vi "Copy Definition.vi"(6 "Source Linked List ID":string, 7 "Sink Linked List ID":string, 8 "error in (no error)":errorcluster, 10 "Sink Parent Linked List ID":string, 11 "Linked List in":refnum<class "Linked List.lvclass">) -> (0 "error out":errorcluster, 3 "Linked List out":refnum<class "Linked List.lvclass">)   [LabVIEW 2017, in "Linked Lists.lvlib" / "Linked List.lvclass"]
uses:
  <vilib>/gpm_packages/@cs/linked-list/Source/Linked List/Linked List/Linked List.lvclass
  <vilib>/gpm_packages/@cs/linked-list/Source/Linked List/Linked List Definition/Linked List Definition.lvclass
  <vilib>/gpm_packages/@cs/linked-list/Source/Linked List/Linked List/Linked List.lvclass/Linked List.ctl
  <vilib>/gpm_packages/@cs/lookup-table/Source/LookupTable/LookupTable.lvclass/LookupTable.ctl
  fc44c7f0-5a9e-40d2-b54b-4ea944ea955e.vi
  566d1f49-e8c0-4e88-a1ce-2ed4a1a2aa01.vi
  d013bb3b-877c-4562-b0e2-39ea021f3923.vi
  <vilib>/gpm_packages/@cs/lookup-table/Source/LookupTable/Read Table Reference.vi
  fc44c7f0-5a9e-40d2-b54b-4ea944ea955e.vi/5b75dade-0515-45f6-8903-5eeabbbc6241.vi
  566d1f49-e8c0-4e88-a1ce-2ed4a1a2aa01.vi/ac60371e-ed5d-4c42-9a6c-bb762d6fad24.vi
  d013bb3b-877c-4562-b0e2-39ea021f3923.vi/90c978a3-e6f6-4f1a-b781-e83e293bed5b.vi
  <vilib>/gpm_packages/@cs/lookup-table/Source/LookupTable/LookupTable.lvclass
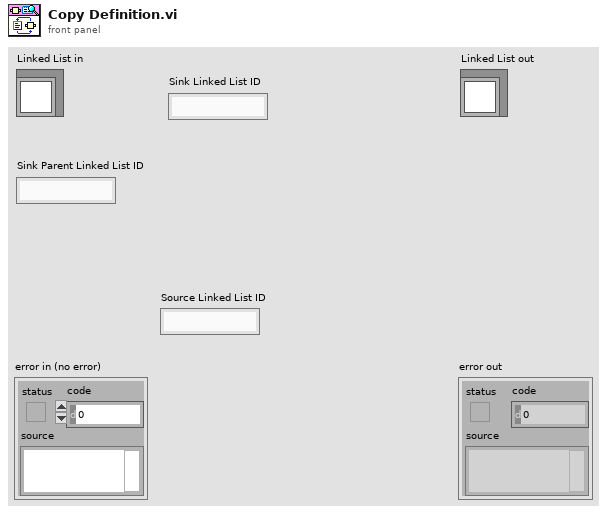
[diagram p1: front panel]
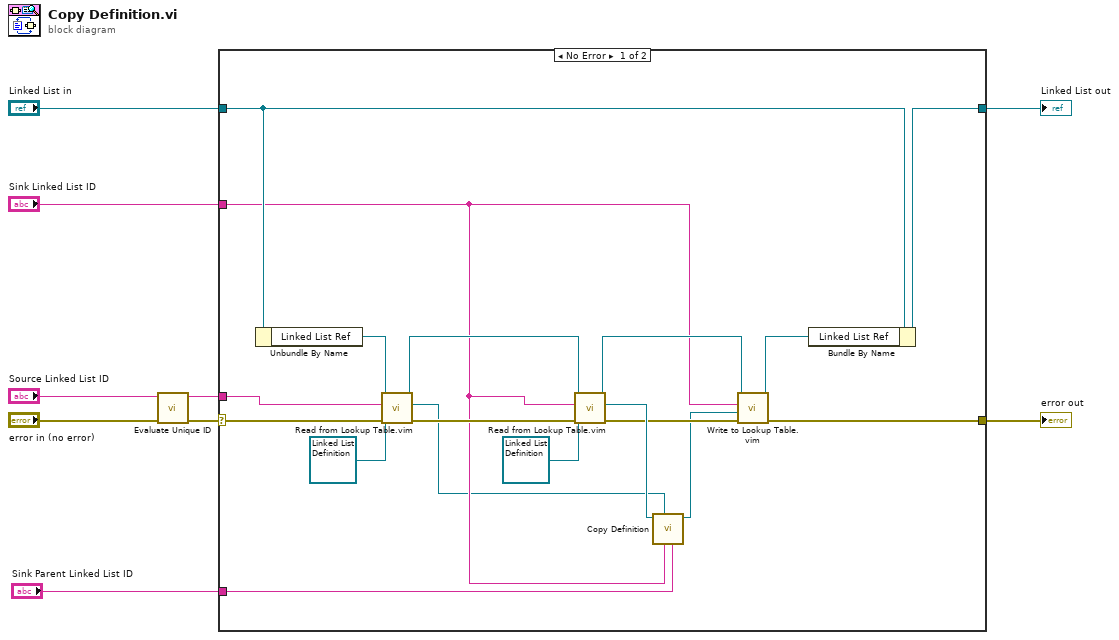
[diagram p0: block diagram]
diagram:
  n1 = call <vilib>:"Evaluate Unique ID.vi"("error in (no error)"="error in (no error)", "Unique ID"="Source Linked List ID") -> ("error out"=w5:errorcluster, "Unique ID Out"=w3:string)  [unwired: 8 in]
  n2 = case shown="No Error" w5 {
    selector: w5 -> [w25 w29]
    tunnel: [w13 w29] -> w9
    tunnel: [w22 w28] -> w7
    tunnel: "Linked List in" -> [w20 w28]
    tunnel: w3 -> [w24 _]
    tunnel: "Sink Linked List ID" -> [w12 _]
    tunnel: "Sink Parent Linked List ID" -> [w17 _]
    frame No Error {
      n3 = Unbundle By Name(w20) -> ("Linked List Ref"=w27:refnum<data-value>)
      n4 = call "Read from Lookup Table.vim"("error in (no error)"=w25, "Type"=refnum<class "Linked List Definition.lvclass"> refnum ("Linked List.lvlib:Linked List Definition.lvclass"), "Item Name"=w24, "LookupTable Reference"=w27) -> ("error out"=w21:errorcluster, "Value"=w10:refnum<class "Linked List Definition.lvclass">, "LookupTable Reference Out"=w19:refnum<data-value>)  [unwired: 4 in, 1 out]
      n5 = call "Read from Lookup Table.vim"("error in (no error)"=w21, "Type"=refnum<class "Linked List Definition.lvclass"> refnum ("Linked List.lvlib:Linked List Definition.lvclass"), "Item Name"=w12, "LookupTable Reference"=w19) -> ("error out"=w14:errorcluster, "Value"=w18:refnum<class "Linked List Definition.lvclass">, "LookupTable Reference Out"=w16:refnum<data-value>)  [unwired: 4 in, 1 out]
      n6 = call <vilib>:"Copy Definition.vi"("Parent Linked List ID"=w17, "Linked List ID"=w12, "Linked List Definition Source"=w10, "Linked List Definition in"=w18) -> ("Linked List Definition out"=w11:refnum<class "Linked List Definition.lvclass">)  [unwired: 7 in]
      n7 = call "Write to Lookup Table.vim"("error in (no error)"=w14, "Item"=w11, "Item Name"=w12, "LookupTable Reference"=w16) -> ("error out"=w13:errorcluster, "LookupTable Reference Out"=w15:refnum<data-value>)  [unwired: 5 in, 1 out]
      n8 = Bundle By Name(cluster=w20, "Linked List Ref"=w15) -> (w22:refnum<class "Linked List.lvclass">)
    }
    frame Error {
    }
  }
  "error out" <- w9
  "Linked List out" <- w7
